vi "String to time stamp.vi"(8 "error in (no error)":errorcluster, 11 "Data In":string[][](array[string])) -> (0 "error out":errorcluster, 3 "Time Stamp Out":timestamp[](array[timestamp])=[timestamp(3597589800 s since 1904-01-01), timestamp(3597589800 s since 1904-01-01), timestamp(3597589800 s since 1904-01-01), timestamp(3597589800 s since 1904-01-01), timestamp(3597589800 s since 1904-01-01), timestamp(3597589800 s since 1904-01-01)] format="%<%X>T")   [LabVIEW 2017]
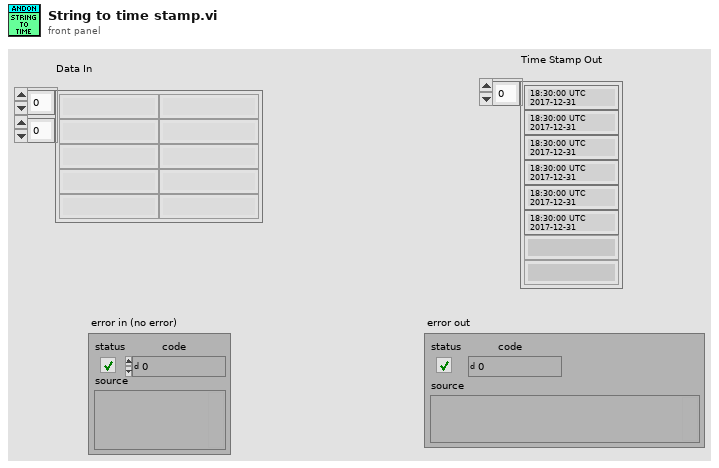
[diagram p1: front panel]
types:
  T1 = cluster{"second":i32, "minute":i32, "hour":i32, "day of month":i32, "month":i32, "year":i32, "day of week":i32, "day of year":i32, "is DST":i32}
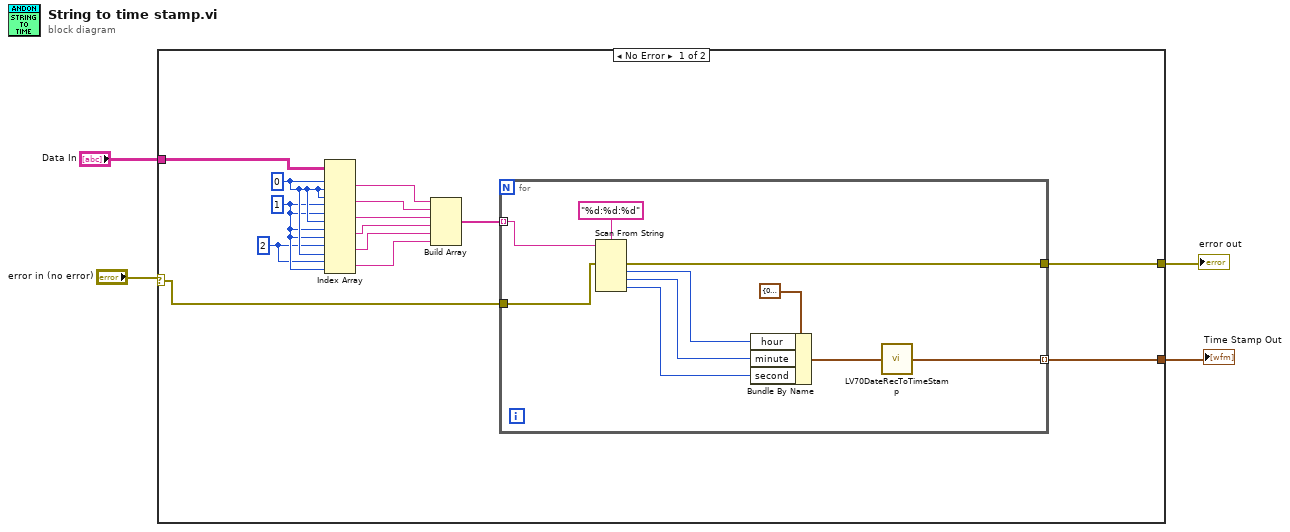
[diagram p0: block diagram]
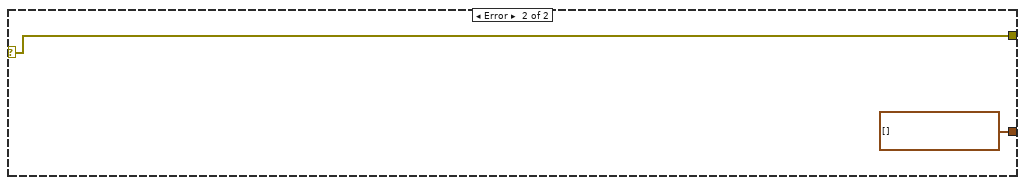
[diagram p2: hidden frame]
diagram:
  n1 = case shown="No Error" "error in (no error)" {
    selector: "error in (no error)" -> [w8 w30]
    tunnel: [w7 w30] -> w3
    tunnel: [w5 timestamp[] []] -> w1
    tunnel: "Data In" -> [w6 _]
    frame No Error {
      w16 = 2 ("disabled index (row)")
      w17 = 1 ("index (col)")
      w18 = 0 ("index (row)")
      n2 = Index Array(array=w6, index (row) #1=w18, index (col) #1=w18, index (row) #2=w18, index (col) #2=w17, index (row) #3=w17, index (col) #3=w18, index (row) #4=w17, index (col) #4=w17, index (row) #5=w16, index (col) #5=w18, index (row) #6=w16, index (col) #6=w17) -> (element #1=w15:string, element #2=w14:string, element #3=w13:string, element #4=w12:string, element #5=w11:string, element #6=w10:string)
      n3 = Build Array(w15, w14, w13, w12, w11, w10) -> (w9:string[])
      n4 = for {
        tunnel: w9 -> [w28] mode=indexing
        tunnel: w8 -> [w21]
        tunnel: [w20] -> w7
        tunnel: [w19] -> w5 mode=indexing
        n5 = Scan From String(format string="%d:%d:%d", input string=w28, error in=w21) -> (error out=w20:errorcluster, output 1=w24:i32, output 2=w23:i32, output 3=w22:i32)  [unwired: 4 in, 2 out]
        n6 = Bundle By Name(cluster=T1 {"second"=0, "minute"=0, "hour"=0, "day of month"=1, "month"=1, "year"=2018, "day of week"=0, "day of year"=0, "is DST"=0} ("date time rec"), "hour"=w24, "minute"=w23, "second"=w22) -> (w26:T1)
        n7 = call <vilib>:"LV70DateRecToTimeStamp.vi"("date time rec"=w26) -> ("Time Stamp"=w19:timestamp)
      }
    }
    frame Error {
    }
  }
  "error out" <- w3
  "Time Stamp Out" <- w1
